vi "Realtime Data.vi"(5 "New Data":dbl[][](array[numeric]), 6 "Enum":enum16{"Init", "Read", "Write"}(ring), 10 "Realtime Data Ref":refnum<vi>) -> (4 "New Data":dbl[][](array[numeric]))   [LabVIEW 2019]
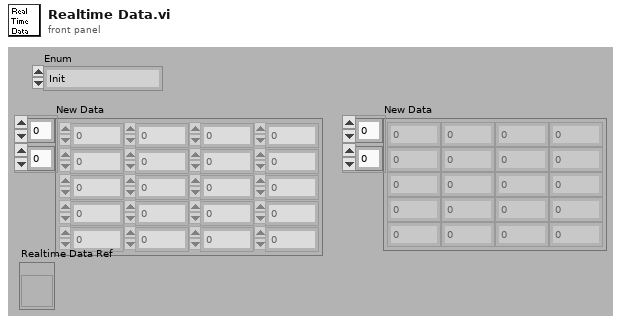
[diagram p1: front panel]
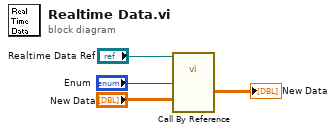
[diagram p0: block diagram]
diagram:
  n1 = call-by-ref "?"(reference="Realtime Data Ref", "New Data"="New Data", "Enum"="Enum") -> ("New Data"=→"New Data":dbl[][])  [unwired: 1 in, 2 out]
